vi "告警码字段定义.vi"(11 "告警代码":u16) -> (1 "故障详情":string, 2 "通用告警信息":string, 3 "字符串":string)   [LabVIEW 2016, in "斯坦道CODMn新电路板.lvlib"]
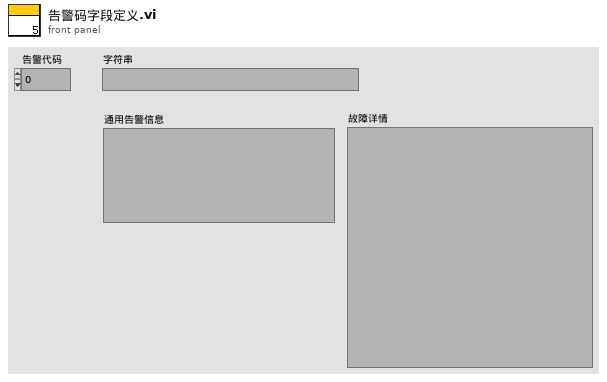
[diagram p1: front panel]
types:
  T1 = cluster{"系统时间":timestamp, "工作状态":u16, "测量模式":enum16{"待机", "连续模式", "周期模式", "定点模式", "受控模式", "手动模式"}, "告警代码":u16, "故障代码":u16, "日志代码":u16, "软件版本":u16, "A":sgl, "B":sgl, "K":sgl, "当前滴定数":sgl, "T":sgl, "H":sgl, "id":u16, "flowid":u16, "量程":u16, "加热实时温度":sgl, "当前ORP值":sgl, "运行时间":sgl, "当前步骤剩余时间":sgl, "结束滴定数":sgl, "注射泵保温温度":sgl}
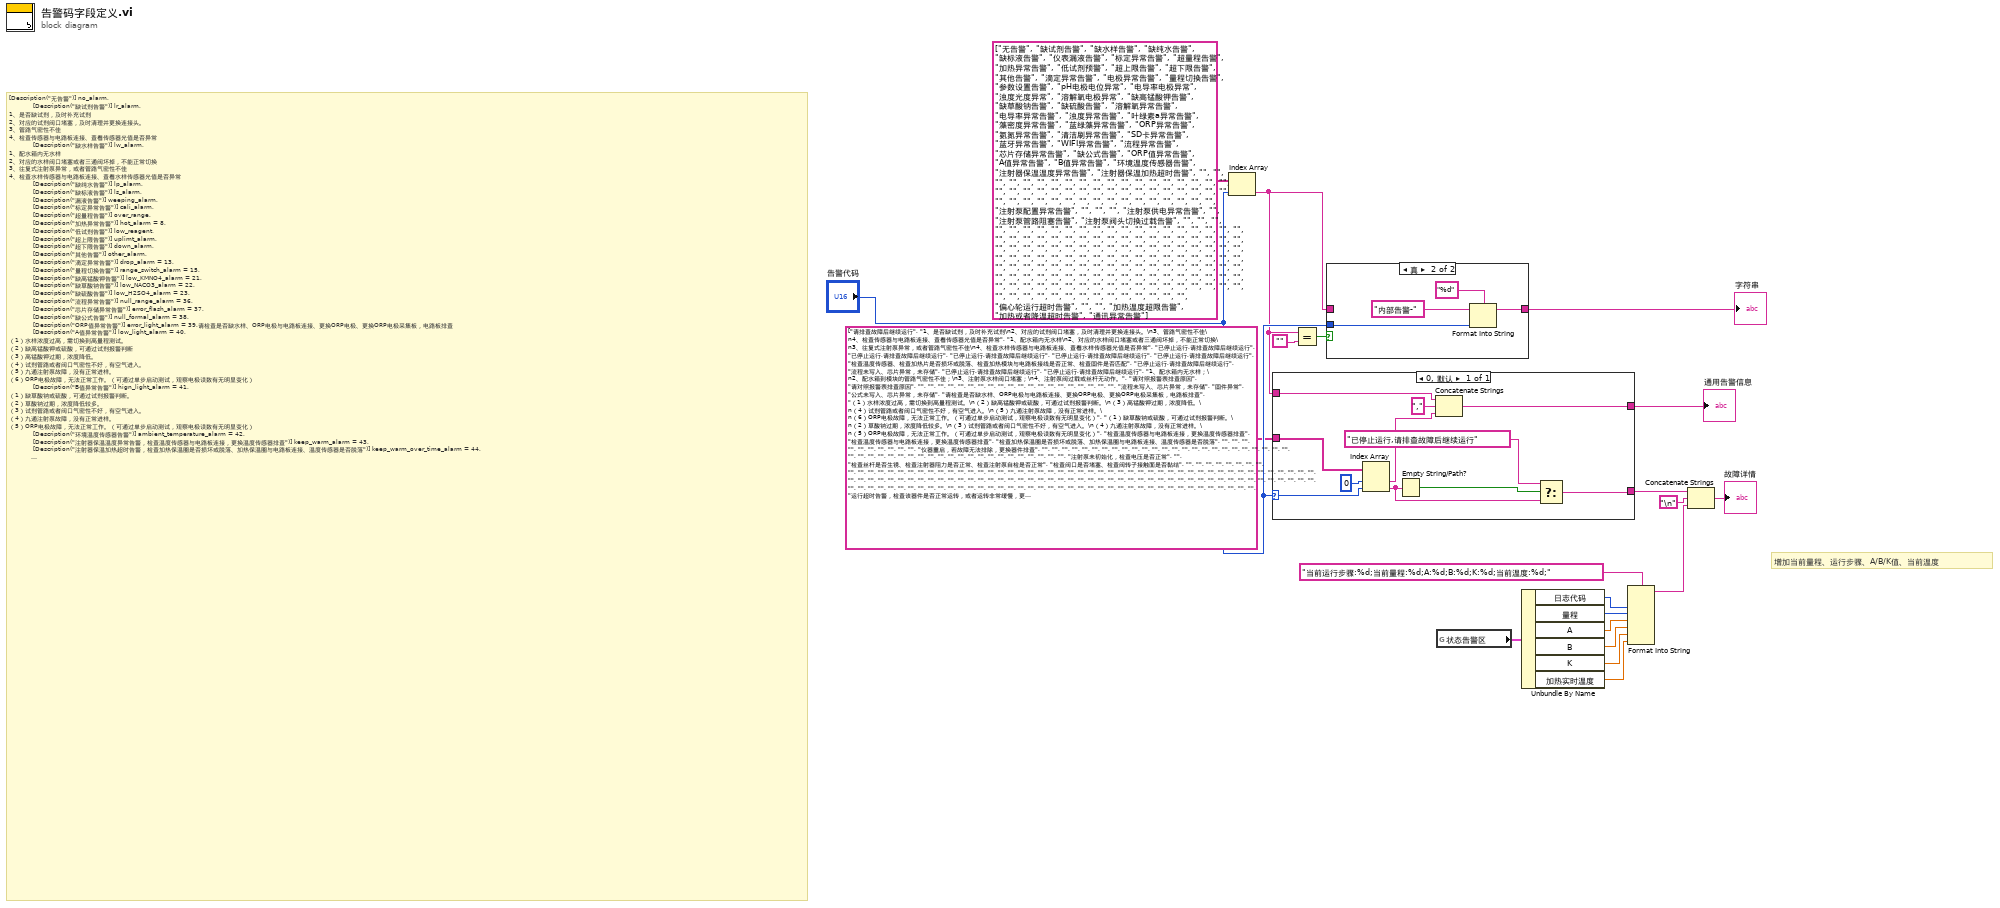
[diagram p0: block diagram]
diagram:
  # "增加当前量程、运行步骤、A/B/K值、当前温度"
  # "[Description(\"无告警\")] no_alarm,\n            [Description(\"缺试剂告警\")] lr_alarm,\n1、是否缺试剂，及时补充试剂\n2、对应的试剂阀口堵塞，及时清理并更换连接头。\n3、管路气密性不佳\n4、检查传感器与电路板连接、查看传感器光值是否异常\n            [Description(\"缺水样告警\")] lw_alarm,\n1、配水箱内无水样\n2、对应的水样阀口堵塞或者三通阀坏掉，不能正常切换\n3、往复式注射泵异常，或者管路气密性不佳\n4、检查水样传感器与电路板连接、查看水样传感器光值是否异常\n            [Description(\"缺纯水告警\")] lp_alarm,\n            [Description(\"缺标液告警\")] ls_alarm,\n            [Description(\"漏液告警\")] weeping_alarm,\n            [Description(\"标定异常告警\")] cali_alarm,\n            [Description(\"超量程告警\")] over_range,\n            [Description(\"加热异常告警\")] hot_alarm = 8,\n            [Description(\"低试剂告警\")] low_reagent,\n            [Description(\"超上限告警\")] uplimt_alarm,\n            [Description(\"超下限告警\")] down_alarm,\n            [Description(\"其他告警\")] other_alarm,\n            [Description(\"滴定异常告警\")] drop_alarm = 13,\n            [Description(\"量程切换告警\")] range_switch_alarm = 15,\n            [Description(\"缺高锰酸钾告警\")] low_KMNO4_alarm = 21,\n            [Description(\"缺草酸钠告警\")] low_NACO3_alarm = 22,\n            [Description(\"缺硫酸告警\")] low_H2SO4_alarm = 23,\n            [Description(\"流程异常告警\")] null_range_alarm = 36,\n            [Description(\"芯片存储异常告警\")] error_flash_alarm = 37,\n            [Description(\"缺公式告警\")] null_formal_alarm = 38,\n            [Description(\"ORP值异常告警\")] error_light_alarm = 39,请检查是否缺水样、ORP电极与电路板连接、更换ORP电极、更换ORP电极采集板，电路板排查\n            [Description(\"A值异常告警\")] low_light_alarm = 40,\n（1）水样浓度过高，需切换到高量程测试。\n（2）缺高锰酸钾或硫酸，可通过试剂报警判断\n（3）高锰酸钾过期，浓度降低。\n（4）试剂管路或者阀口气密性不好，有空气进入。\n（5）九通注射泵故障，没有正常进样。\n（6）ORP电极故障，无法正常工作。（可通过单步启动测试，观察电极读数有无明显变化）\n            [Description(\"B值异常告警\")] hign_light_alarm = 41,\n（1）缺草酸钠或硫酸，可通过试剂报警判断。\n（2）草酸钠过期，浓度降低较多。\n（3）试剂管路或者阀口气密性不好，有空气进入。\n（4）九通注射泵故障，没有正常进样。\n（5）ORP电极故障，无法正常工作。（可通过单步启动测试，观察电极读数有无明显变化）\n            [Description(\"环境温度传感器告警\")] ambient_temperature_alarm = 42,\n            [Description(\"注射器保温温度异常告警，检查温度传感器与电路板连接，更换温度传感器排查\")] keep_warm_alarm = 43,\n            [Description(\"注射器保温加热超时告警，检查加热保温圈是否损坏或脱落、加热保温圈与电路板连接、温度传感器是否脱落\")] keep_warm_over_time_alarm = 44,\n            [Description(\"注射泵未初始化，检查电压是否正常\")] pump_not_Initialized_alarm = 103,\n            [Description(\"检查丝杆是否生锈、检查注射器阻力是否正常、检查注射泵自检是否正常\")] pump_Plunger_Overload_alarm = 105,\n            [Description(\"检查阀口是否堵塞、检查阀转子接触面是否黏结\")] pump_Valve_Overload_alarm = 106,\n            [Description(\"运行超时告警，检查该器件是否正常运转，或者运转非常缓慢，更换器件排查\")] pump_re_over_time_alarm = 250,\n            [Description(\"加热温度超限告警，检查温度传感器与电路板连接、检查是否缺水样\")] hot_temp_alarm = 253,\n            [Description(\"加热或者降温超时告警，检查加热圈是否损坏或脱落、加热圈与电路板连接、温度传感器是否脱落\")] hot_over_time_alarm = 254,\n            [Description(\"通讯异常告警，检查该器件与电路板通讯，重新插拔端子排查\")] communicate_alarm = 255,"
  n1 = Index Array(array=string[] ["无告警", "缺试剂告警", "缺水样告警", "缺纯水告警", "缺标液告警", "仪表漏液告警", "标定异常告警", "超量程告警", "加热异常告警", "低试剂预警", "超上限告警", "超下限告警", "其他告警", "滴定异常告警", "电极异常告警", "量程切换告警", "参数设置告警", "pH电极电位异常", "电导率电极异常", "浊度光度异常", "溶解氧电极异常", "缺高锰酸钾告警", "缺草酸钠告警", "缺硫酸告警", "溶解氧异常告警", "电导率异常告警", "浊度异常告警", "叶绿素a异常告警", "藻密度异常告警", "蓝绿藻异常告警", "ORP异常告警", "氨氮异常告警", "清洁刷异常告警", "SD卡异常告警", "蓝牙异常告警", "WIFI异常告警", "流程异常告警", "芯片存储异常告警", "缺公式告警", "ORP值异常告警", "A值异常告警", "B值异常告警", "环境温度传感器告警", "注射器保温温度异常告警", "注射器保温加热超时告警", "", "", "", "", "", "", "", "", "", "", "", "", "", "", "", "", "", "", "", "", "", "", "", "", "", "", "", "", "", "", "", "", "", "", "", "", "", "", "", "", "", "", "", "", "", "", "", "", "", "", "", "", "", "", "注射泵配置异常告警", "", "", "", "注射泵供电异常告警", "", "注射泵管路阻塞告警", "注射泵阀头切换过载告警", "", "", "", "", "", "", "", "", "", "", "", "", "", "", "", "", "", "", "", "", "", "", "", "", "", "", "", "", "", "", "", "", "", "", "", "", "", "", "", "", "", "", "", "", "", "", "", "", "", "", "", "", "", "", "", "", "", "", "", "", "", "", "", "", "", "", "", "", "", "", "", "", "", "", "", "", "", "", "", "", "", "", "", "", "", "", "", "", "", "", "", "", "", "", "", "", "", "", "", "", "", "", "", "", "", "", "", "", "", "", "", "", "", "", "", "", "", "", "", "", "", "", "", "", "", "", "", "", "", "", "", "", "", "", "", "", "", "", "", "", "", "", "", "偏心轮运行超时告警", "", "", "加热温度超限告警", "加热或者降温超时告警", "通讯异常告警"], index="告警代码") -> (element=w13:string)
  n2 = case shown="0, 默认" "告警代码" {
    selector: "告警代码" -> [w29]
    tunnel: string[] ["请排查故障后继续运行", "1、是否缺试剂，及时补充试剂\n2、对应的试剂阀口堵塞，及时清理并更换连接头。\n3、管路气密性不佳\n4、检查传感器与电路板连接、查看传感器光值是否异常", "1、配水箱内无水样\n2、对应的水样阀口堵塞或者三通阀坏掉，不能正常切换\n3、往复式注射泵异常，或者管路气密性不佳\n4、检查水样传感器与电路板连接、查看水样传感器光值是否异常", "已停止运行,请排查故障后继续运行", "已停止运行,请排查故障后继续运行", "已停止运行,请排查故障后继续运行", "已停止运行,请排查故障后继续运行", "已停止运行,请排查故障后继续运行", "检查温度传感器、检查加热片是否损坏或脱落、检查加热模块与电路板接线是否正常、检查固件是否匹配", "已停止运行,请排查故障后继续运行", "流程未写入、芯片异常，未存储", "已停止运行,请排查故障后继续运行", "已停止运行,请排查故障后继续运行", "1、配水箱内无水样；\n2、配水箱到模块的管路气密性不佳；\n3、注射泵水样阀口堵塞；\n4、注射泵阀过载或丝杆无动作。", "请对照报警表排查原因", "请对照报警表排查原因", "", "", "", "", "", "", "", "", "", "", "", "", "", "", "", "", "", "", "", "", "流程未写入、芯片异常，未存储", "固件异常", "公式未写入、芯片异常，未存储", "请检查是否缺水样、ORP电极与电路板连接、更换ORP电极、更换ORP电极采集板，电路板排查", "（1）水样浓度过高，需切换到高量程测试。\n（2）缺高锰酸钾或硫酸，可通过试剂报警判断。\n（3）高锰酸钾过期，浓度降低。\n（4）试剂管路或者阀口气密性不好，有空气进入。\n（5）九通注射泵故障，没有正常进样。\n（6）ORP电极故障，无法正常工作。（可通过单步启动测试，观察电极读数有无明显变化）", "（1）缺草酸钠或硫酸，可通过试剂报警判断。\n（2）草酸钠过期，浓度降低较多。\n（3）试剂管路或者阀口气密性不好，有空气进入。\n（4）九通注射泵故障，没有正常进样。\n（5）ORP电极故障，无法正常工作。（可通过单步启动测试，观察电极读数有无明显变化）", "检查温度传感器与电路板连接，更换温度传感器排查", "检查温度传感器与电路板连接，更换温度传感器排查", "检查加热保温圈是否损坏或脱落、加热保温圈与电路板连接、温度传感器是否脱落", "", "", "", "", "", "", "", "", "", "", "仪器重启，若故障无法排除，更换器件排查", "", "", "", "", "", "", "", "", "", "", "", "", "", "", "", "", "", "", "", "", "", "", "", "", "", "", "", "", "", "", "", "", "", "", "", "", "", "", "", "", "", "", "", "", "", "", "", "注射泵未初始化，检查电压是否正常", "", "检查丝杆是否生锈、检查注射器阻力是否正常、检查注射泵自检是否正常", "检查阀口是否堵塞、检查阀转子接触面是否黏结", "", "", "", "", "", "", "", "", "", "", "", "", "", "", "", "", "", "", "", "", "", "", "", "", "", "", "", "", "", "", "", "", "", "", "", "", "", "", "", "", "", "", "", "", "", "", "", "", "", "", "", "", "", "", "", "", "", "", "", "", "", "", "", "", "", "", "", "", "", "", "", "", "", "", "", "", "", "", "", "", "", "", "", "", "", "", "", "", "", "", "", "", "", "", "", "", "", "", "", "", "", "", "", "", "", "", "", "", "", "", "", "", "", "", "", "", "", "", "", "", "", "", "", "", "", "", "", "", "", "", "", "", "", "", "", "", "", "", "", "", "", "", "", "运行超时告警，检查该器件是否正常运转，或者运转非常缓慢，更换器件排查", "", "", "检查温度传感器与电路板连接、检查是否缺水样", "检查加热圈是否损坏或脱落、加热圈与电路板连接、温度传感器是否脱落", "通讯异常告警，检查该器件与电路板通讯，重新插拔端子排查"] -> [w27]
    tunnel: [w25] -> w14
    tunnel: [w21] -> w4
    tunnel: w13 -> [w28]
    frame 0, Default {
      n3 = Index Array(array=w27, index #1=0 ("索引"), index #2=w29) -> (element #1=w26:string, element #2=w22:string)
      n4 = Empty String/Path?(string/path=w22) -> (empty?=w24:bool)
      n5 = Concatenate Strings(w28, "," ("字符串"), w26) -> (w25:string)
      n6 = Select(t="已停止运行,请排查故障后继续运行" ("工作状态"), s=w24, f=w22) -> (s? t:f=w21:string)
    }
  }
  "通用告警信息" <- w14
  n7 = Equal?(x=w13, y="") -> (x = y?=w18:bool)
  n8 = case shown="真" w18 {
    tunnel: [w32 w34] -> w17
    tunnel: w13 -> [w32 _]
    tunnel: "告警代码" -> [_ w33]
    frame False {
    }
    frame True {
      n9 = Format Into String(format string="%d" ("格式字符串"), initial string="内部告警-" ("工作状态"), w33) -> (resulting string=w34:string)  [unwired: 1 in, 1 out]
    }
  }
  "字符串" <- w17
  n10 = global read "VARCODMn全局变量.vi" "状态告警区"() -> (w12:T1)
  n11 = Unbundle By Name(w12) -> ("日志代码"=w10:u16, "量程"=w9:u16, "A"=w8:sgl, "B"=w7:sgl, "K"=w6:sgl, "加热实时温度"=w5:sgl)
  n12 = Format Into String(format string="当前运行步骤:%d;当前量程:%d;A:%d;B:%d;K:%d;当前温度:%d;" ("格式字符串"), w10, w9, w8, w7, w6, w5) -> (resulting string=w1:string)  [unwired: 2 in, 1 out]
  n13 = Concatenate Strings(w4, "\n", w1) -> (→"故障详情":string)
